vi "Lab_2_subVI_tank_1_Ashish.vi"(8 "hss,1":dbl, 9 "A1":dbl, 10 "a1":dbl, 11 "U":dbl) -> (2 "height tank1":dbl, 3 "H1":dbl)   [LabVIEW 2020]
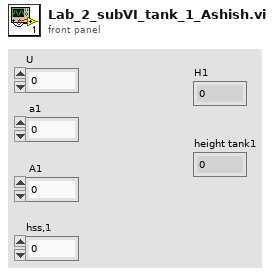
[diagram p1: front panel]
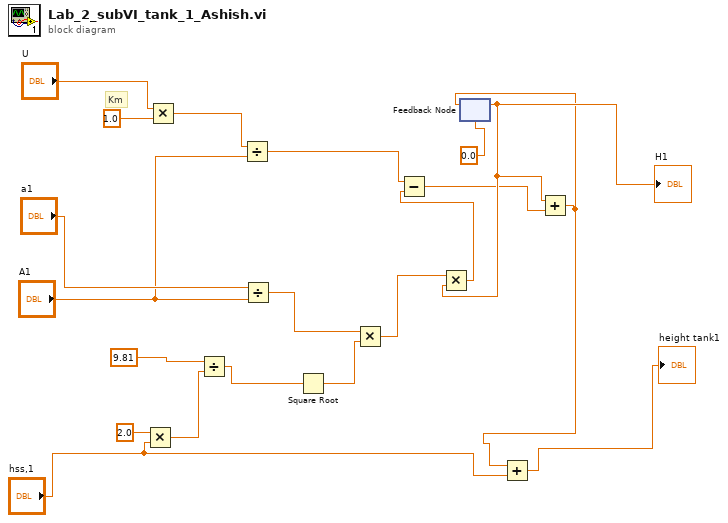
[diagram p0: block diagram]
diagram:
  # "Km"
  n1 = Multiply(x=2.0, y="hss,1") -> (x*y=w12:dbl)
  n2 = Multiply(x="U", y=1.0 ("Km")) -> (x*y=w18:dbl)
  n3 = Divide(x=9.81, y=w12) -> (x/y=w11:dbl)
  n4 = Divide(x=w18, y="A1") -> (x/y=w9:dbl)
  n5 = Divide(x="a1", y="A1") -> (x/y=w15:dbl)
  n6 = Square Root(x=w11) -> (sqrt(x)=w10:dbl)
  n7 = Multiply(x=w15, y=w10) -> (x*y=w8:dbl)
  n8 = feedback #1(0.0 ("y")) -> (w5:dbl)
  "H1" <- w5
  n9 = Multiply(x=w8, y=w5) -> (x*y=w7:dbl)
  n10 = Subtract(x=w9, y=w7) -> (x-y=w4:dbl)
  n11 = Add(x=w5, y=w4) -> (x+y=w3:dbl)
  n12 = feedback-in #1(w3) -> ()
  n13 = Add(x=w3, y="hss,1") -> (x+y=→"height tank1":dbl)
